vi "create_ramp.vi"(7 "channel":T1, 8 "error in (no error)":errorcluster, 9 "end color":cluster{dbl, dbl, dbl, dbl}(slide) scale=1e-10..255.0, 10 "start color":cluster{dbl, dbl, dbl, dbl}(slide) scale=1e-10..255.0, 11 "ColorOverlay in":refnum<class "ColorOverlay.lvclass">) -> (0 "error out":errorcluster, 2 "ramp array out":u32[](array[numeric]), 3 "ColorOverlay out":refnum<class "ColorOverlay.lvclass">, 4 "ramp array out correct dec":u32[](array[numeric]), 5 "ramp array out corrected hex":u32[](array[numeric]))   [LabVIEW 2010, in "ColorOverlay.lvclass"]
uses:
  ColorOverlay.lvclass
  enum_color_channel.ctl
  ColorOverlay.lvclass/ColorOverlay.ctl
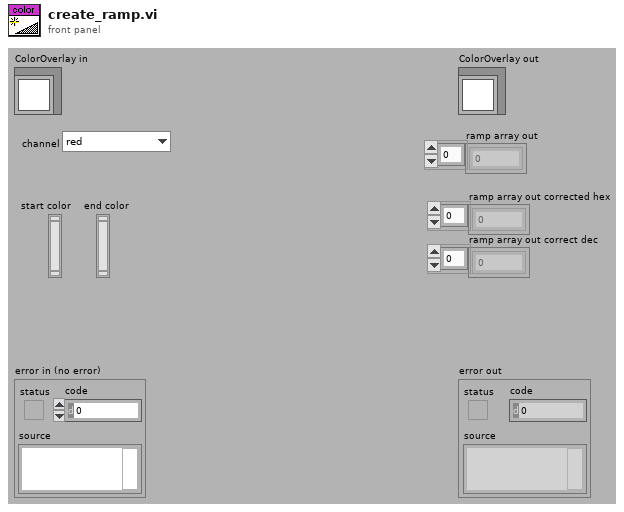
[diagram p1: front panel]
types:
  T1 = typedef "ColorOverlay.lvclass/enum_color_channel.ctl" = enum16{"red", "green", "blue", "gray"}
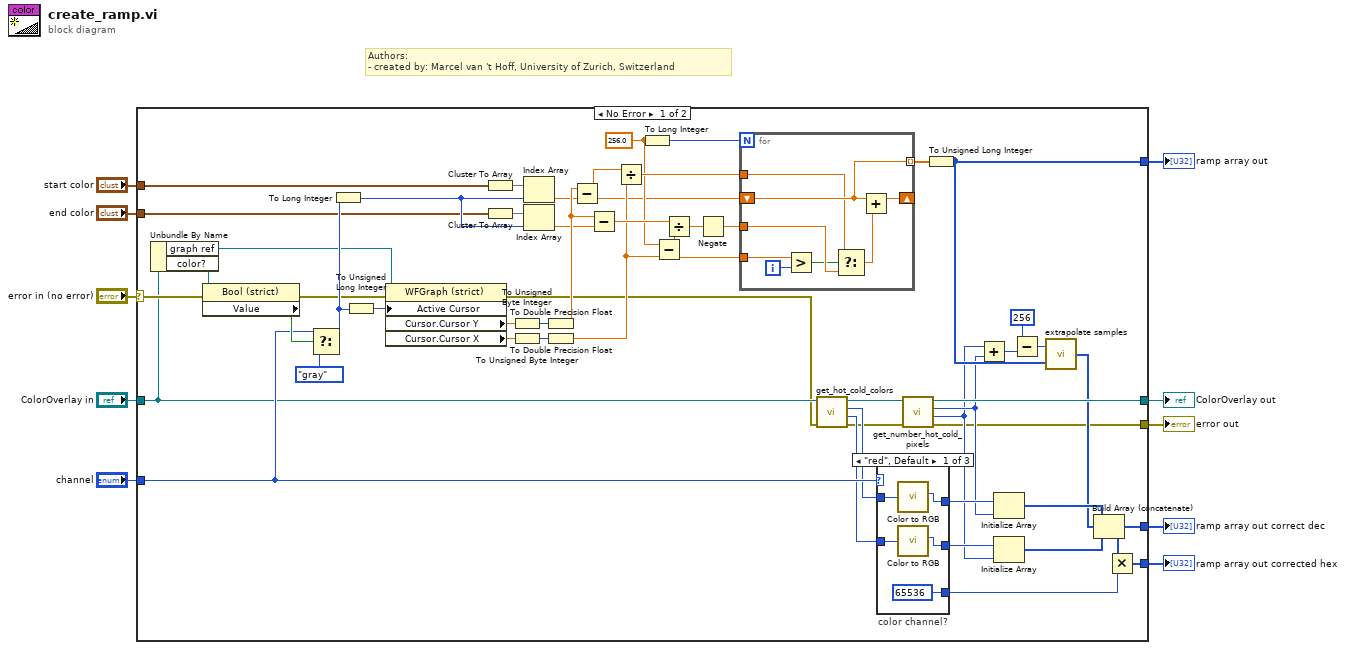
[diagram p0: block diagram]
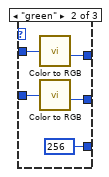
[diagram p2: hidden frame]
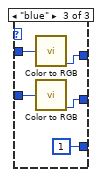
[diagram p3: hidden frame]
diagram:
  # "Authors: \n- created by: Marcel van 't Hoff, University of Zurich, Switzerland"
  n1 = case shown="No Error" "error in (no error)" {
    selector: "error in (no error)" -> [w53 w88]
    tunnel: [w13 w88] -> w9
    tunnel: [w23 w87] -> w7
    tunnel: "ColorOverlay in" -> [w18 w87]
    tunnel: [w32 _] -> w6
    tunnel: "start color" -> [w50 _]
    tunnel: "end color" -> [w49 _]
    tunnel: "channel" -> [w31 _]
    tunnel: [w17 _] -> w2
    tunnel: [w15 _] -> w1
    frame No Error {
      w37 = 256.0
      n2 = Unbundle By Name(w18) -> ("graph ref"=w55:refnum<vi>, "color?"=w54:refnum<vi>)
      n3 = property class="Bool (strict)"(reference=w54, error in=w53) -> (error out=w51:errorcluster, "Value"=w52:bool)  [unwired: 1 out]
      n4 = Select(t=w31, s=w52, f=enum_color_channel."gray" ("channel")) -> (s? t:f=w61:T1)
      n5 = To Long Integer(number=w61) -> (32bit integer=w59:i32)
      n6 = To Unsigned Long Integer(number=w61) -> (unsigned 32bit integer=w57:u32)
      n7 = property class="WFGraph (strict)"(reference=w55, error in=w51, "Active Cursor"=w57) -> (error out=w14:errorcluster, "Cursor.Cursor Y"=w62:dbl, "Cursor.Cursor X"=w63:dbl)  [unwired: 1 out]
      n8 = Cluster To Array(cluster=w50) -> (array=w56:dbl[])
      n9 = Cluster To Array(cluster=w49) -> (array=w58:dbl[])
      n10 = To Unsigned Byte Integer(number=w62) -> (unsigned 8bit integer=w47:u8)
      n11 = To Unsigned Byte Integer(number=w63) -> (unsigned 8bit integer=w46:u8)
      n12 = Index Array(array=w56, index=w59) -> (element=w11:dbl)
      n13 = Index Array(array=w58, index=w59) -> (element=w12:dbl)
      n14 = To Double Precision Float(number=w47) -> (double precision float=w45:dbl)
      n15 = To Double Precision Float(number=w46) -> (double precision float=w39:dbl)
      n16 = Subtract(x=w45, y=w11) -> (x-y=w44:dbl)
      n17 = Subtract(x=w45, y=w12) -> (x-y=w43:dbl)
      n18 = Divide(x=w44, y=w39) -> (x/y=w38:dbl)
      n19 = To Long Integer(number=w37) -> (32bit integer=w36:i32)
      n20 = Subtract(x=w37, y=w39) -> (x-y=w40:dbl)
      n21 = Divide(x=w43, y=w40) -> (x/y=w42:dbl)
      n22 = Negate(x=w42) -> (-x=w41:dbl)
      n23 = for {
        N: w36 -> [_]
        shift-right: [w86] -> _
        shift-left: w11 -> [w85]
        tunnel: w38 -> [w82]
        tunnel: w41 -> [w83]
        tunnel: [w85] -> w48 mode=indexing
        tunnel: w39 -> [w79]
        i -> [w84]
        n24 = Greater?(x=w79, y=w84) -> (0:w80:bool)
        n25 = Select(t=w82, s=w80, f=w83) -> (s? t:f=w81:dbl)
        n26 = Add(x=w85, y=w81) -> (x+y=w86:dbl)
      }
      n27 = call-dynamic "get_hot_cold_colors.vi"("error in (no error)"=w14, "ColorOverlay in"=w18) -> ("error out"=w19:errorcluster, "color upper limit"=w29:u32, "color lower limit"=w30:u32, "ColorOverlay out"=w24:refnum<class "ColorOverlay.lvclass">)  [unwired: 6 in]
      n28 = case "color channel?" shown="\"red\", Default" w31 {
        tunnel: w30 -> [w68 w73 w78]
        tunnel: [w67 w70 w76] -> w26
        tunnel: w29 -> [w66 w72 w77]
        tunnel: [w65 w71 w75] -> w25
        tunnel: [u32 65536 u32 256 u32 1] -> w16
        frame "red", Default {
          n29 = call <vilib>:"Color to RGB.vi"("Color"=w68) -> ("R"=w67:u8)  [unwired: 3 out]
          n30 = call <vilib>:"Color to RGB.vi"("Color"=w66) -> ("R"=w65:u8)  [unwired: 3 out]
        }
        frame "green" {
          n31 = call <vilib>:"Color to RGB.vi"("Color"=w73) -> ("G"=w70:u8)  [unwired: 3 out]
          n32 = call <vilib>:"Color to RGB.vi"("Color"=w72) -> ("G"=w71:u8)  [unwired: 3 out]
        }
        frame "blue" {
          n33 = call <vilib>:"Color to RGB.vi"("Color"=w78) -> ("B"=w76:u8)  [unwired: 3 out]
          n34 = call <vilib>:"Color to RGB.vi"("Color"=w77) -> ("B"=w75:u8)  [unwired: 3 out]
        }
      }
      n35 = call-dynamic "get_number_hot_cold_pixels.vi"("error in (no error)"=w19, "ColorOverlay in"=w24) -> ("error out"=w13:errorcluster, "# hot pixels"=w20:i32, "# cold pixels"=w21:i32, "ColorOverlay out"=w23:refnum<class "ColorOverlay.lvclass">)  [unwired: 6 in]
      n36 = To Unsigned Long Integer(number=w48) -> (unsigned 32bit integer=w32:u32[])
      n37 = Add(x=w20, y=w21) -> (x+y=w35:i32)
      n38 = Initialize Array(w26, w21) -> (w27:u8[])
      n39 = Initialize Array(w25, w20) -> (w28:u8[])
      n40 = Subtract(x=256, y=w35) -> (x-y=w33:i32)
      n41 = call "extrapolate samples.vi"("ramp array in"=w32, "new sample number"=w33) -> ("extrapolated array out"=w22:u32[])
      n42 = Build Array (concatenate)(w27, w22, w28) -> (w15:u32[])
      n43 = Multiply(x=w15, y=w16) -> (x*y=w17:u32[])
    }
    frame Error {
    }
  }
  "error out" <- w9
  "ColorOverlay out" <- w7
  "ramp array out" <- w6
  "ramp array out corrected hex" <- w2
  "ramp array out correct dec" <- w1
